vi "SpinnerMotorsValue.vi"() -> ()   [LabVIEW 2016]
panel:
  out "SpinnerMotorsValue":dbl
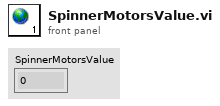
[diagram p1: front panel]
diagram:
